vi "API-Reference to DVR.vi"(1 "API-Reference in":refnum<k1>) -> (0 "Data Value Reference out":refnum<data-value>)   [LabVIEW 2018, in "Actor.lvclass"]
uses:
  Actor.lvclass
  API-Data.ctl
  Stopped.ctl
  Event-References.ctl
  Stop.ctl
  Launched.ctl
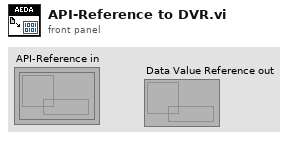
[diagram p1: front panel]
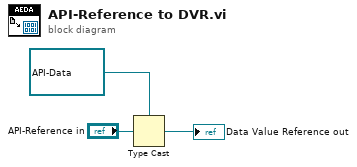
[diagram p0: block diagram]
diagram:
  n1 = Type Cast(type=refnum<data-value> refnum ("API_DVR"), x="API-Reference in") -> (*(type *) &x=→"Data Value Reference out":refnum<data-value>)
